vi "AlliGator FMB Event to String.vi"(5 "Add Ellipsis (T)":bool=TRUE, 8 "FMB Q Event":T1=enum."Idle") -> (2 "String":string)   [LabVIEW 2021, in "AlliGator Fit Method Benchmark.lvlib"]
doc: "Converts <B>AlliGator Q Event</B> enum to the corresponding string."
uses:
  AlliGator Fit Method Benchmark.lvlib
  Notebook/AlliGator Notebook.lvlib
  AlliGator FMB Q Event List.ctl
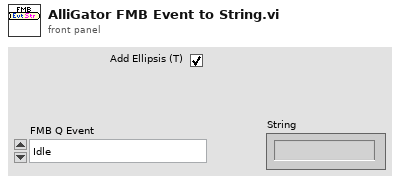
[diagram p1: front panel]
types:
  T1 = typedef "AlliGator Fit Method Benchmark.lvlib/AlliGator FMB Q Event List.ctl" = enum16{"Update Script Simulation Parameters", "Idle", "Run Simulation", "Update Histograms", "Graph Event", "Show Selected Decay", "Export Results", "Update # Processors Used", "Check Baseline", "Run Script", "End Script", "Init", "Abort", "Quit"}
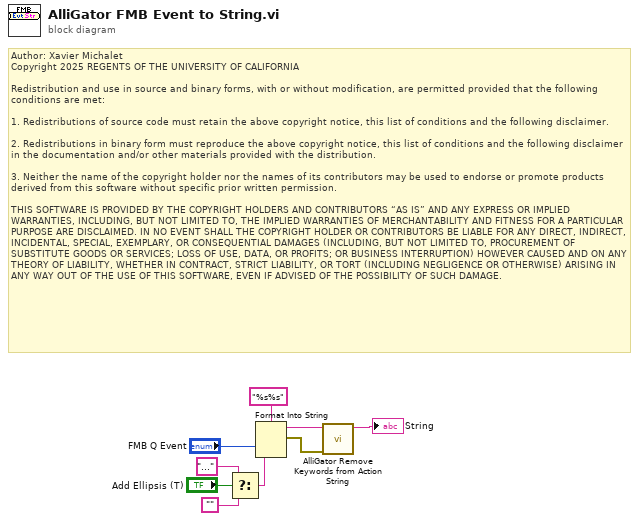
[diagram p0: block diagram]
diagram:
  # "Author: Xavier Michalet\nCopyright 2025 REGENTS OF THE UNIVERSITY OF CALIFORNIA\n\nRedistribution and use in source and binary forms, with or without modification, are permitted provided that the following conditions are met:\n\n1. Redistributions of source code must retain the above copyright notice, this list of conditions and the following disclaimer.\n\n2. Redistributions in binary form must reproduce the above copyright notice, this list of conditions and the following disclaimer in the documentation and/or other materials provided with the distribution.\n\n3. Neither the name of the copyright holder nor the names of its contributors may be used to endorse or promote products derived from this software without specific prior written permission.\n\nTHIS SOFTWARE IS PROVIDED BY THE COPYRIGHT HOLDERS AND CONTRIBUTORS “AS IS” AND ANY EXPRESS OR IMPLIED WARRANTIES, INCLUDING, BUT NOT LIMITED TO, THE IMPLIED WARRANTIES OF MERCHANTABILITY AND FITNESS FOR A PARTICULAR PURPOSE ARE DISCLAIMED. IN NO EVENT SHALL THE COPYRIGHT HOLDER OR CONTRIBUTORS BE LIABLE FOR ANY DIRECT, INDIRECT, INCIDENTAL, SPECIAL, EXEMPLARY, OR CONSEQUENTIAL DAMAGES (INCLUDING, BUT NOT LIMITED TO, PROCUREMENT OF SUBSTITUTE GOODS OR SERVICES; LOSS OF USE, DATA, OR PROFITS; OR BUSINESS INTERRUPTION) HOWEVER CAUSED AND ON ANY THEORY OF LIABILITY, WHETHER IN CONTRACT, STRICT LIABILITY, OR TORT (INCLUDING NEGLIGENCE OR OTHERWISE) ARISING IN ANY WAY OUT OF THE USE OF THIS SOFTWARE, EVEN IF ADVISED OF THE POSSIBILITY OF SUCH DAMAGE."
  n1 = Select(t="..." ("format string"), s="Add Ellipsis (T)", f="") -> (s? t:f=w5:string)
  n2 = Format Into String(format string="%s%s", "FMB Q Event", w5) -> (resulting string=w3:string, error out=w2:errorcluster)  [unwired: 2 in]
  n3 = call "AlliGator Remove Keywords from Action String.vi"("error in (no error)"=w2, "String"=w3) -> ("String w/o keywords"=→"String":string)  [unwired: 8 in, 1 out]
